vi "Get Subsystem Variables.vi"(8 "error in (no error)":errorcluster, 11 "Subsystem URL":refnum<k21>) -> (0 "error out":errorcluster, 2 "Variable Names":string[](array[string]), 3 "Variable URLs":refnum<k21>[](array[refnum]), 4 "Subsystem Name":string)   [LabVIEW 2024]
doc: "Gets the I/O variables in a subsystem from the shared variable engine."
uses:
  <resource>/objmgr/ni.var.rc
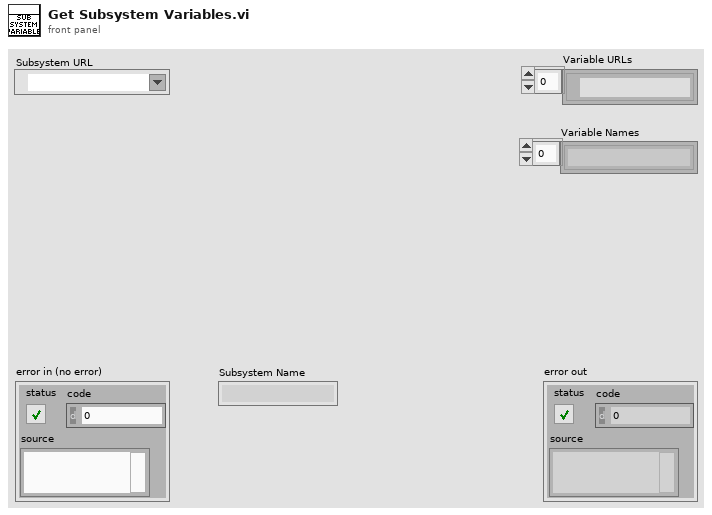
[diagram p1: front panel]
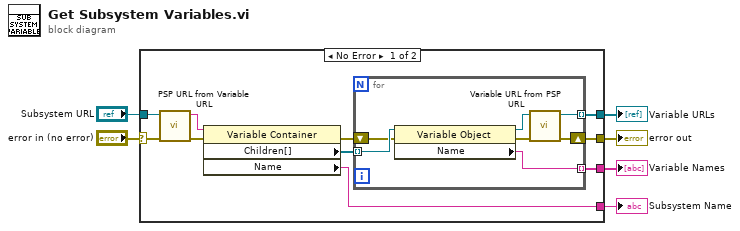
[diagram p0: block diagram]
diagram:
  n1 = case shown="No Error" "error in (no error)" {
    selector: "error in (no error)" -> [w11 w24]
    tunnel: [w16 w24] -> w6
    tunnel: "Subsystem URL" -> [w10 _]
    tunnel: [w8 _] -> w4
    tunnel: [w7 _] -> w3
    tunnel: [w9 _] -> w2
    frame No Error {
      n2 = call "PSP URL from Variable URL.vi"("error in (no error)"=w11, "Shared Variable URL"=w10) -> ("error out"=w12:errorcluster, "PSP URL"=w13:string)  [unwired: 8 in]
      n3 = property class="Variable Container"(reference=w13, error in=w12) -> (error out=w14:errorcluster, "Children[]"=w15:refnum<k21>[], "Name"=w9:string)  [unwired: 1 out]
      n4 = for {
        tunnel: w15 -> [w23] mode=indexing
        shift-right: [w20] -> w16
        shift-left: w14 -> [w22]
        tunnel: [w18] -> w8 mode=indexing
        tunnel: [w17] -> w7 mode=indexing
        n5 = property class="Variable Object"(reference=w23, error in=w22) -> (reference out=w19:refnum<k21>, error out=w21:errorcluster, "Name"=w17:string)
        n6 = call "Variable URL from PSP URL.vi"("error in (no error)"=w21, "PSP URL"=w19) -> ("error out"=w20:errorcluster, "Shared Variable URL"=w18:refnum<k21>)  [unwired: 8 in]
      }
    }
    frame Error {
    }
  }
  "error out" <- w6
  "Variable URLs" <- w4
  "Variable Names" <- w3
  "Subsystem Name" <- w2
